vi "DeviceQuery.vi"(4 "error in (no error)":errorcluster, 5 "Command":string, 6 "DeviceKey In":string, 7 "USBLib In":refnum<k24>) -> (0 "error out":errorcluster, 1 "Response":string, 2 "DeviceKey Out":string, 3 "USBLib Out":refnum<k24>)   [LabVIEW 2009]
uses:
  C:/Samples/LabVIEW/UseDeviceKey/LabVIEW 2009/UseDeviceKey (with Device VIs)/UsbDllWrap.dll
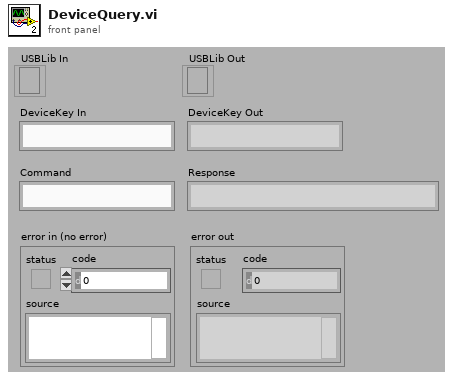
[diagram p1: front panel]
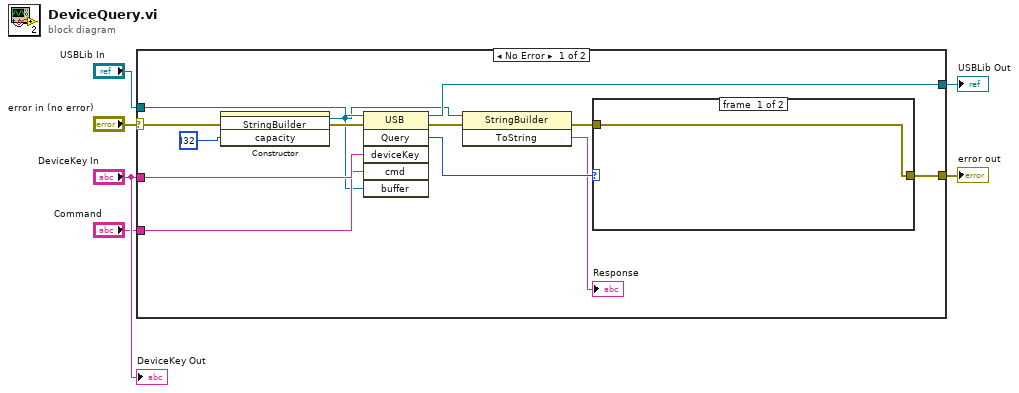
[diagram p0: block diagram]
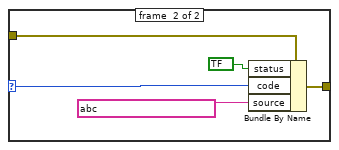
[diagram p2: hidden frame]
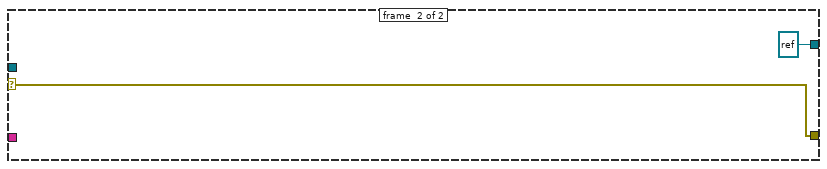
[diagram p3: hidden frame]
diagram:
  n1 = case shown="No Error" "error in (no error)" {
    selector: "error in (no error)" -> [w14 w27]
    tunnel: [w8 w27] -> w5
    tunnel: "DeviceKey In" -> [w19 _]
    tunnel: "Command" -> [w18 _]
    tunnel: "USBLib In" -> [w17 _]
    tunnel: [w16 refnum<k24> ? ("USBLib In")] -> w1
    frame #0 {
      n2 = constructor class="StringBuilder"(error in=w14, "capacity"=i32 ?) -> (reference out=w11:refnum<k24>, error out=w13:errorcluster)  [unwired: 2 in, 2 out]
      n3 = invoke class="USB" method="Query"(reference=w17, error in=w13, "deviceKey"=w19, "cmd"=w18, "buffer"=w11) -> (reference out=w16:refnum<k24>, error out=w12:errorcluster, "Query"=w10:i32)  [unwired: 1 in, 3 out]
      n4 = invoke class="StringBuilder" method="ToString"(reference=w11, error in=w12) -> (error out=w9:errorcluster, "ToString"=→"Response":string)  [unwired: 1 in, 1 out]
      n5 = case shown="1, Default" w10 {
        selector: w10 -> [_ w21]
        tunnel: w9 -> [w20 w23]
        tunnel: [w20 w22] -> w8
        frame #0 {
        }
        frame #1 {
          n6 = Bundle By Name(cluster=w23, "status"=bool ?, "code"=w21, "source"=string ?) -> (w22:errorcluster)
        }
      }
    }
    frame #1 {
    }
  }
  "error out" <- w5
  "USBLib Out" <- w1
  "DeviceKey Out" <- "DeviceKey In"
